vi "CRC32.vi"(11 "CRC32Settings":T1={"DataFIFO"="GyroCRCDataFIFO", "CalculateFIFO"="GyroCRCCalculateFIFO", "CRCFIFO"="GyroCRCFIFO"}) -> ()   [LabVIEW 2016]
uses:
  CRC32Settings.ctl
  CRC32Data.ctl
  CRC32States.ctl
  <vilib>/Platform/TimedLoop/XDataNode/timing_clust.ctl
  <vilib>/Platform/TimedLoop/XDataNode/nitl_modes.ctl
  <vilib>/Platform/TimedLoop/XDataNode/wakeup.ctl
  <vilib>/rvi/Emulation/niFpgaSctlEmulationGetInTimedLoop.vi
  <vilib>/rvi/Emulation/niFpgaEmulationReportErrorSimple.vi
  <vilib>/rvi/Emulation/niFpgaGetClockAttributes.vi
  <vilib>/rvi/Emulation/niFpgaCriticalErrorInLSC.vi
  <vilib>/rvi/DataTransferAndStorage/Container/Common/niFpgaContainerExecOnDevCompGetState.vi
  <vilib>/rvi/Emulation/niFpgaEmulationIsFPGAContextNoSignature.vi
  <vilib>/rvi/errors/niFpgaSetErrorForExecOnDevCompSimple.vi
  <vilib>/rvi/eio/common/nirviEmuReportErrorAndStop.vi
  <vilib>/rvi/DataTransferAndStorage/Container/Common/niFpgaContainerGetUniqueNameForEmu.vi
  <vilib>/rvi/FIFO/Fifo_Resource/nirvififoEmulationSetSize.vi
  <vilib>/rvi/FIFO/Fifo_Resource/nirviFifoEmulationQueueMgr.vi
  <instcachedir>/0/nirviFifoEmulationQueueMgr_E5CAEC123FF24DC58D834DCA3CDAA9B5.lvgen/nirviFifoEmulationQueueMgr_E5CAEC123FF24DC58D834DCA3CDAA9B5_009.vi
  <vilib>/rvi/FIFO/Fifo_Resource/nirvififoEmulationDetermineInputValidOut.vi
  <vilib>/rvi/FIFO/Fifo_Resource/nirvififoEmulationCreateLock.vi
  <vilib>/rvi/Emulation/niFpgaProcessEmulError.vi
  <vilib>/rvi/FIFO/Fifo_Resource/nirvififoEmulationObtainLock.vi
  <vilib>/rvi/FIFO/Fifo_Resource/nirvififoEmulationReleaseLock.vi
  <vilib>/rvi/occurrence/nirviWaitOnOccurrenceBase.vi
  <vilib>/rvi/errors/nirviReportUnexpectedCaseInternalError.vi
  <vilib>/rvi/errors/nirviReportUnexpectedCaseInternalError (U32).vi
  <vilib>/Utility/error.llb/Clear Errors.vi
  <vilib>/rvi/interface/RandomDataEmulation/niFpgaRandomDataHandleErrors.vi
  <instcachedir>/0/nirviFifoEmulationQueueMgr_E5CAEC123FF24DC58D834DCA3CDAA9B5.lvgen/nirviFifoEmulationQueueMgr_E5CAEC123FF24DC58D834DCA3CDAA9B5_004.vi
  <instcachedir>/0/nirviFifoEmulationQueueMgr_E5CAEC123FF24DC58D834DCA3CDAA9B5.lvgen/nirviFifoEmulationQueueMgr_E5CAEC123FF24DC58D834DCA3CDAA9B5_006.vi
  <vilib>/Platform/TimedLoop/XDataNode/XDataNode.xnode
  <vilib>/rvi/DataTransferAndStorage/Container/XNode/niFpgaContainer.xnode
  <vilib>/rvi/FIFO/Fifo_Resource/niFpgaFifoEmulationRefIn.vi
  <vilib>/Platform/TimedLoop/XDataNode/XDNodeRunTimeDep.lvlib
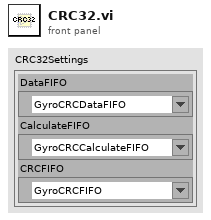
[diagram p1: front panel]
types:
  T1 = typedef "CRC32Settings.ctl" = cluster{"DataFIFO":refnum<k21>, "CalculateFIFO":refnum<k21>, "CRCFIFO":refnum<k21>}
  T2 = typedef "CRC32Data.ctl" = cluster{"State":T3, "Bit":u8, "CRC":u32, "Word":u8}
  T3 = typedef "CRC32States.ctl" = enum16{"WaitForData", "ProcessData", "CheckForPublish", "PublishCRC"}
  T4 = typedef "XDNodeRunTimeDep.lvlib/timing_clust.ctl" = cluster{"Expected End [f-1]":u64, "Actual End [f-1]":u64, "Finished Late? [f-1]":bool, "Expected End [i-1]":u64, "Actual End [i-1]":u64, "Finished Late? [i-1]":bool, "Expected Start [i]":u64, "Actual Start [i]":u64, "Expected Start [f]":u64, "Actual Start [f]":u64, "Source Name":string, "Structure Name":string, "Period":i64, "Deadline":i64, "Offset":i64, "Start":i64, "Priority":i32, "Timeout":i32, "Mode":T5, "Wakeup Reason":T6, "Error":errorcluster, "Source Type":string, "Secondary Source Type":string, "Global End Time":u64, "Global Start Time":u64, "Frame Duration":u64, "Iteration Duration":u64, "Assigned CPU":i32, "I/O Scan Engine Mode":u32}
  T5 = typedef "XDNodeRunTimeDep.lvlib/nitl_modes.ctl" = enum32{"No Change", "Process missed periods, maintain original phase", "Discard missed periods, maintain original phase", "Process missed periods, ignore original phase", "Discard missed periods, ignore original phase"}
  T6 = typedef "XDNodeRunTimeDep.lvlib/wakeup.ctl" = enum32{"Normal", "Aborted", "Asynchronous wakeup", "Timing source error", "Timed loop error", "Timeout"}
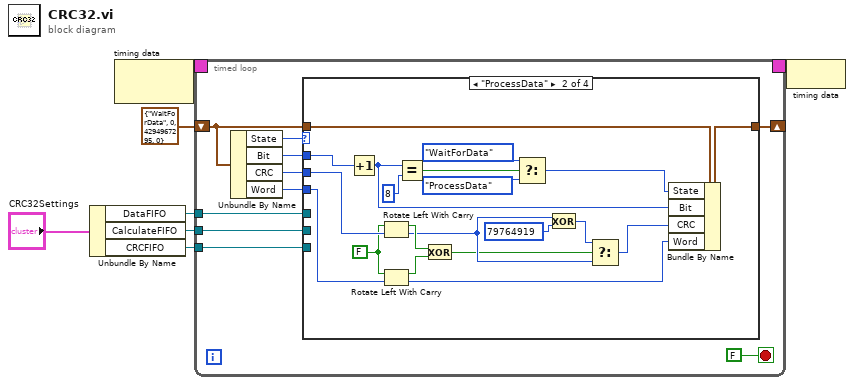
[diagram p0: block diagram]
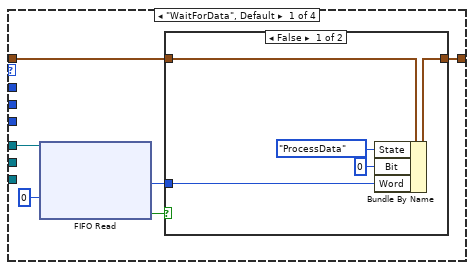
[diagram p2: hidden frame]
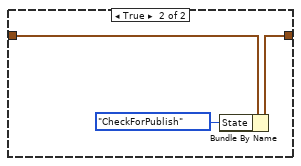
[diagram p3: hidden frame]
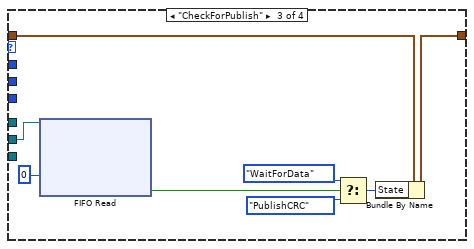
[diagram p4: hidden frame]
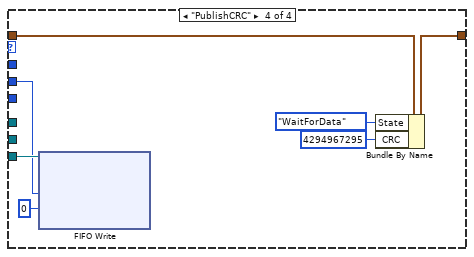
[diagram p5: hidden frame]
diagram:
  n1 = Unbundle By Name("CRC32Settings") -> ("DataFIFO"=w4:refnum<k21>, "CalculateFIFO"=w3:refnum<k21>, "CRCFIFO"=w2:refnum<k21>)
  n2 = node-c288() -> (w7:T4)  [unwired: 1 in]
  n3 = timed-loop {
    shift-right: [w16] -> _
    shift-left: T2 {"State"=enum."WaitForData", "Bit"=0, "CRC"=4294967295, "Word"=0} ("CRC32Data") -> [w15]
    timing: w7 -> [_]
    timing-out: [_] -> w6
    tunnel: w4 -> [w13]
    tunnel: w3 -> [w12]
    tunnel: w2 -> [w11]
    stop <- FALSE stop-if-true
    n4 = Unbundle By Name(w15) -> ("State"=w17:T3, "Bit"=w10:u8, "CRC"=w14:u32, "Word"=w8:u8)
    n5 = case shown="\"ProcessData\"" w17 {
      tunnel: [w18 w50 w58 w65] -> w16
      tunnel: w15 -> [w23 w51 w59 w66]
      tunnel: w14 -> [_ w42 _ w62]
      tunnel: w13 -> [w22 _ _ _]
      tunnel: w12 -> [_ _ w57 _]
      tunnel: w11 -> [_ _ _ w63]
      tunnel: w10 -> [_ w49 _ _]
      tunnel: w8 -> [_ w41 _ _]
      frame "WaitForData", Default {
        n6 = xnode ("FIFO Read")("Timeout"=0, "FIFO In"=w22) -> ("Element"=w19:u8, "Timed Out?"=w20:bool)  [unwired: 1 out]
        n7 = case shown="False" w20 {
          tunnel: w23 -> [w28 w31]
          tunnel: w19 -> [w24 _]
          tunnel: [w27 w30] -> w18
          frame False {
            n8 = Bundle By Name(cluster=w28, "State"=CRC32States."ProcessData", "Bit"=u8 0, "Word"=w24) -> (w27:T2)
          }
          frame True {
            n9 = Bundle By Name(cluster=w31, "State"=CRC32States."CheckForPublish") -> (w30:T2)
          }
        }
      }
      frame "ProcessData" {
        w40 = FALSE ("carry")
        n10 = Increment(x=w49) -> (x+1=w43:u8)
        n11 = Rotate Left With Carry(2:w42, 3:w40) -> (0:w34:u32, 1:w38:bool)
        n12 = Rotate Left With Carry(2:w41, 3:w40) -> (0:w37:u8, 1:w39:bool)
        n13 = Equal?(x=w43, y=u8 8) -> (x = y?=w48:bool)
        n14 = Exclusive Or(1:w39, 2:w38) -> (0:w33:bool)
        n15 = Select(t=CRC32States."WaitForData", s=w48, f=CRC32States."ProcessData" ("State")) -> (s? t:f=w45:T3)
        n16 = Exclusive Or(1:u32 79764919, 2:w34) -> (0:w35:u32)
        n17 = Select(t=w35, s=w33, f=w34) -> (s? t:f=w32:u32)
        n18 = Bundle By Name(cluster=w51, "State"=w45, "Bit"=w43, "CRC"=w32, "Word"=w37) -> (w50:T2)
      }
      frame "CheckForPublish" {
        n19 = xnode ("FIFO Read")("Timeout"=0, "FIFO In"=w57) -> ("Timed Out?"=w55:bool)  [unwired: 2 out]
        n20 = Select(t=CRC32States."WaitForData" ("State"), s=w55, f=CRC32States."PublishCRC" ("State")) -> (s? t:f=w52:T3)
        n21 = Bundle By Name(cluster=w59, "State"=w52) -> (w58:T2)
      }
      frame "PublishCRC" {
        n22 = xnode ("FIFO Write")("Element"=w62, "Timeout"=0, "FIFO In"=w63) -> ()  [unwired: 2 out]
        n23 = Bundle By Name(cluster=w66, "State"=CRC32States."WaitForData", "CRC"=u32 4294967295) -> (w65:T2)
      }
    }
  }
  n24 = node-c288(w6) -> ()
